vi "Get Project and Target references.vi"(8 "error in (no error)":errorcluster, 10 "Target Name":string="My Computer", 11 "Project Path":path) -> (0 "error out":errorcluster, 2 "Target refnum":refnum<vi>, 3 "Project refnum":refnum<vi>)   [LabVIEW 2021, in "CIF Build Actions.lvlib"]
uses:
  CIF Build Actions.lvlib
  CIFCore/Common/Typedef/Errors.ctl
  <vilib>/CIF Foundation/CIF Utilities/Errors/Append Error Location.vi
  CIFCore/Common/CIFCoreCommon.lvlib
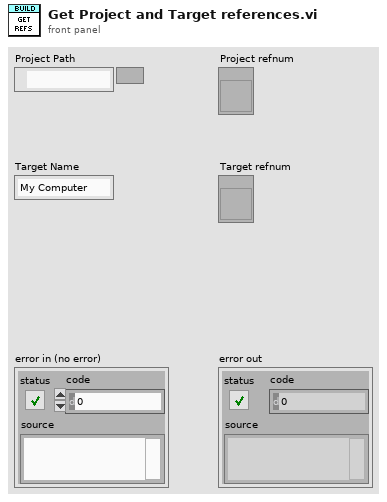
[diagram p1: front panel]
types:
  T1 = typedef "CIFCoreCommon.lvlib/Errors.ctl" = enum16{"Invalid Clock ID", "Long Sleep", "gRPC Server Not Found", "Config Parse", "Timestamp Wrap", "Delayed Execution", "Duplicate Channel", "Missing Channel", "Incorrect Type", "Flatten Error", "Unflatten Data", "Unique Name", "Plugin Not Found", "Plugin Type Not Found", "Plugin Version Not Found", "Manager Not Found", "Numerical Issue", "Time Jump", "Clock ID Match", "Channel Length", "Plugin Connection", "gRPC Server Connection", "PPL Name Match", "Build", "Config Log Parse", "Plugin Load", "UI Subpanel Load", "Python Name", "Invalid Name"}
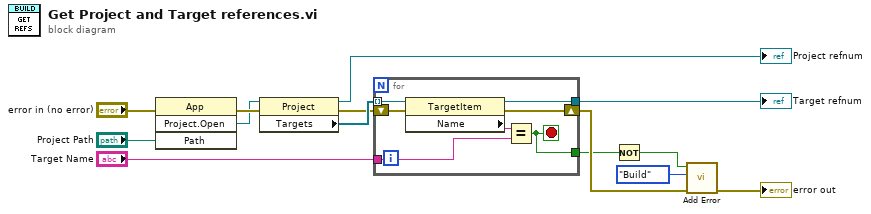
[diagram p0: block diagram]
diagram:
  n1 = invoke class="App" method="Project.Open"(error in="error in (no error)", "Path"="Project Path") -> (error out=w9:errorcluster, "Project:Open"=w7:refnum<vi>)  [unwired: 2 in, 2 out]
  n2 = property class="Project"(reference=w7, error in=w9) -> (reference out=→"Project refnum":refnum<vi>, error out=w6:errorcluster, "Targets"=w10:refnum<vi>[])
  n3 = for {
    tunnel: w10 -> [w21] mode=indexing
    tunnel: "Target Name" -> [w19]
    shift-right: [w17] -> w4
    shift-left: w6 -> [w18]
    tunnel: [w16] -> w8
    tunnel: [w15] -> w2
    stop <- w15 stop-if-true
    n4 = property class="TargetItem"(reference=w21, error in=w18) -> (reference out=w16:refnum<vi>, error out=w17:errorcluster, "Name"=w20:string)
    n5 = Equal?(x=w20, y=w19) -> (x = y?=w15:bool)
  }
  "Target refnum" <- w8
  n6 = Not(x=w2) -> (.not. x?=w1:bool)
  n7 = call "Add Error.vi"("error in (no error)"=w4, "Error"=Errors."Build", "Insert Error"=w1) -> ("error out"=→"error out":errorcluster)  [unwired: 8 in]
